vi "temp_graph.vi"(11 "file path (dialog if empty) in":path) -> (3 "Curva de temperatura":cluster{"Ramp Pattern":dbl[], u32[]}(graph))   [LabVIEW 2021]
uses:
  <vilib>/Analysis/1siggen.llb/Ramp Pattern by Delta.vi
  <vilib>/Analysis/NI_AALBase.lvlib
panel:
  out "Curva de temperatura  2":cluster{"Ramp Pattern":dbl[], u32[]}(graph)
  in  "Array":string[](array[string])
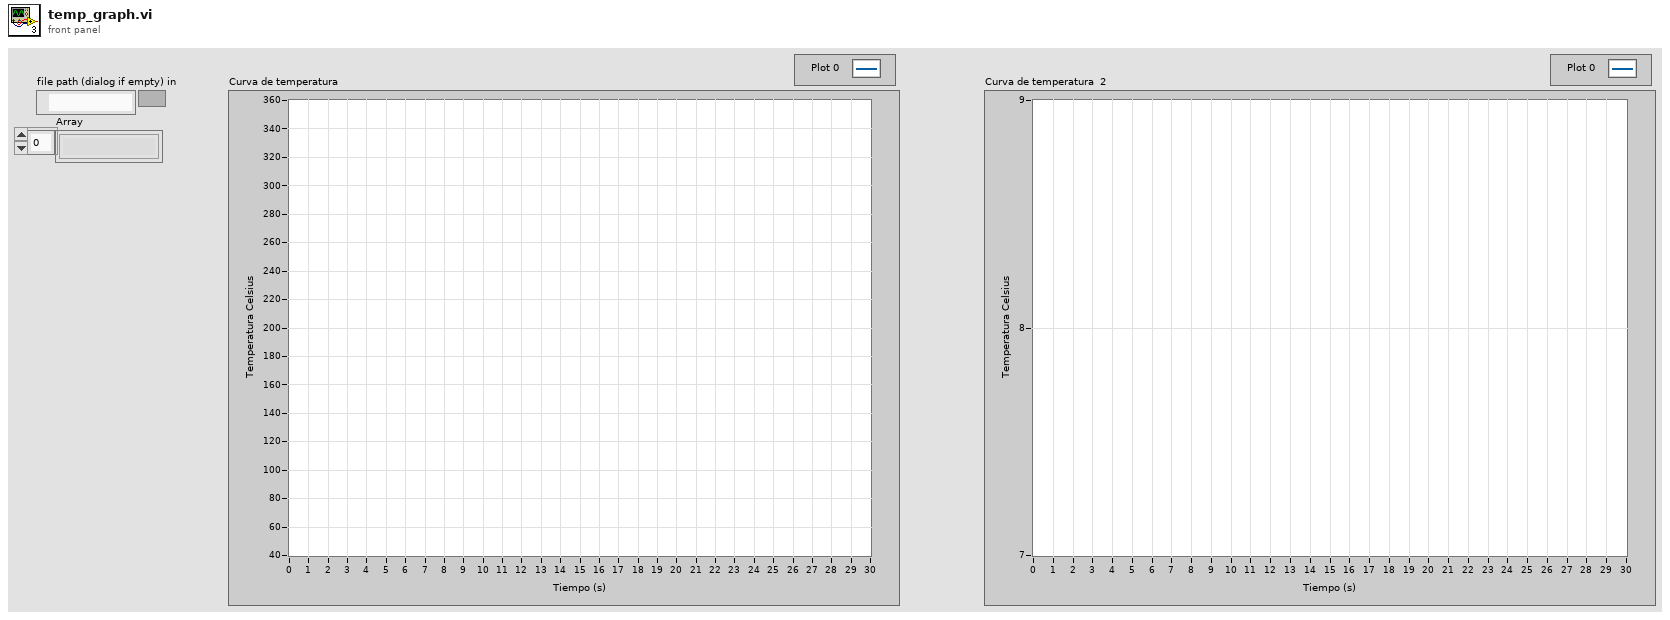
[diagram p1: front panel]
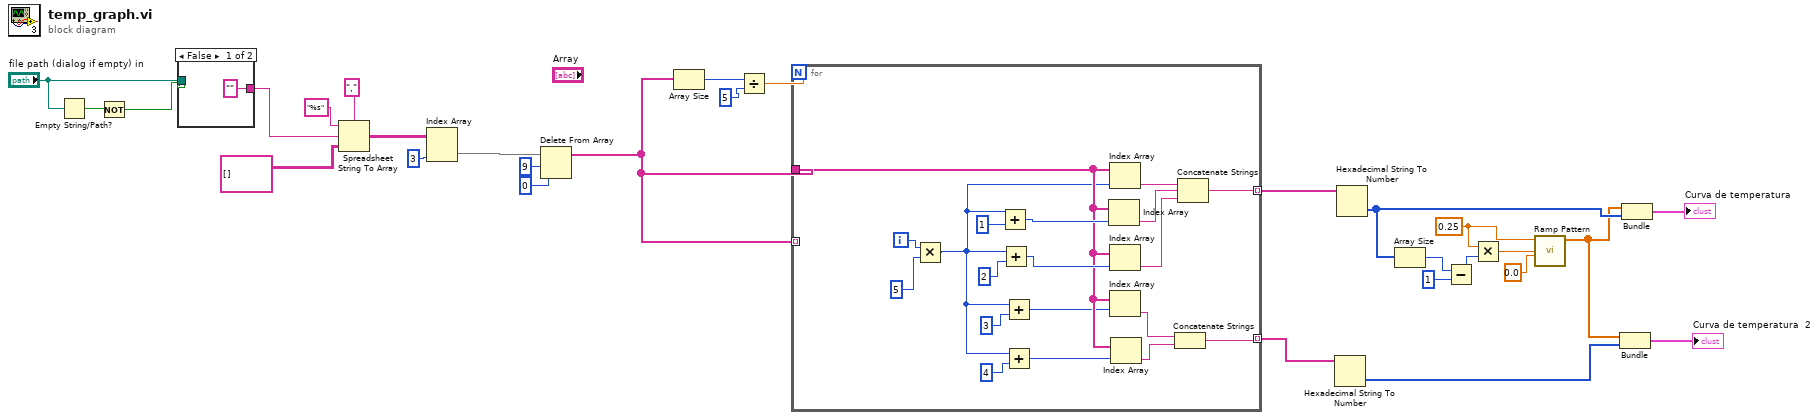
[diagram p0: block diagram]
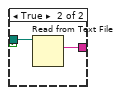
[diagram p2: hidden frame]
diagram:
  w13 = 0.25 ("delta")
  n1 = Empty String/Path?(string/path="file path (dialog if empty) in") -> (empty?=w7:bool)
  n2 = Not(x=w7) -> (.not. x?=w6:bool)
  n3 = case shown="False" w6 {
    tunnel: ["" w32] -> w16
    tunnel: "file path (dialog if empty) in" -> [_ w31]
    frame False {
    }
    frame True {
      n4 = Read from Text File(file (use dialog)=w31) -> (text=w32:string)  [unwired: 3 in, 3 out]
    }
  }
  n5 = Spreadsheet String To Array(delimiter (Tab)=",", format string="%s", spreadsheet string=w16, array type (2D Dbl)=string[][] [] ("Array")) -> (array=w19:string[][])
  n6 = Index Array(array=w19, index (col)=3 ("disabled index (col)")) -> (element=w21:string[])  [unwired: 1 in]
  n7 = Delete From Array(array=w21, length=9, index=0) -> (array with subset deleted=w1:string[])  [unwired: 1 out]
  n8 = Array Size(array=w1) -> (size(s)=w24:i32)
  n9 = Divide(x=w24, y=5) -> (x/y=w26:dbl)
  n10 = for {
    N: w26 -> [_]
    tunnel: w1 -> [_] mode=indexing
    tunnel: w1 -> [w41]
    tunnel: [w48] -> w27 mode=indexing
    tunnel: [w33] -> w5 mode=indexing
    i -> [w43]
    n11 = Multiply(x=w43, y=5) -> (x*y=w40:i32)
    n12 = Add(x=w40, y=1) -> (x+y=w45:i32)
    n13 = Add(x=w40, y=2) -> (x+y=w44:i32)
    n14 = Add(x=w40, y=3) -> (x+y=w37:i32)
    n15 = Add(x=w40, y=4) -> (x+y=w36:i32)
    n16 = Index Array(array=w41, index=w45) -> (element=w50:string)
    n17 = Index Array(array=w41, index=w40) -> (element=w51:string)
    n18 = Index Array(array=w41, index=w44) -> (element=w49:string)
    n19 = Index Array(array=w41, index=w37) -> (element=w35:string)
    n20 = Index Array(array=w41, index=w36) -> (element=w34:string)
    n21 = Concatenate Strings(w35, w34) -> (w33:string)
    n22 = Concatenate Strings(w51, w50, w49) -> (w48:string)
  }
  n23 = Hexadecimal String To Number(string=w5) -> (number=w3:u32[])  [unwired: 2 in, 1 out]
  n24 = Hexadecimal String To Number(string=w27) -> (number=w14:u32[])  [unwired: 2 in, 1 out]
  n25 = Array Size(array=w14) -> (size(s)=w11:i32)
  n26 = Subtract(x=w11, y=1) -> (x-y=w9:i32)
  n27 = Multiply(x=w13, y=w9) -> (x*y=w12:dbl)
  n28 = call-poly <vilib>:"Ramp Pattern.vi"("start"=0.0, "end"=w12, "delta"=w13) -> ("Ramp Pattern"=w4:dbl[])  [unwired: 6 in, 2 out]
  n29 = Bundle("Ramp Pattern"=w4, w3) -> (→"Curva de temperatura  2":cluster{"Ramp Pattern":dbl[], u32[]})  [unwired: 1 in]
  n30 = Bundle("Ramp Pattern"=w4, w14) -> (→"Curva de temperatura":cluster{"Ramp Pattern":dbl[], u32[]})  [unwired: 1 in]
